vi "Real 64 Converter.vi"(7 "Byte Order (Normal)":T1(ring), 9 "Data In":string) -> (1 "Data Array Out":dbl[](array[numeric]))   [LabVIEW 2017, in "Keithley 2600 Series.lvlib"]
doc: "The KE26XXA_Real64Converter accepts REAL64 double precision IEEE-754 binary formatted data returned by printbuffer() and type casts it to an array of floating point numbers used for data analysis. \n\nEach buffer starts with 2330 and ends with 0A. Everything between is data."
uses:
  Keithley 2600 Series.lvlib
panel:
  out "error out":errorcluster
  in  "error in (no error)":errorcluster
  # "(c) 2008 Keithley Instruments, Inc.  ALL RIGHTS RESERVED."
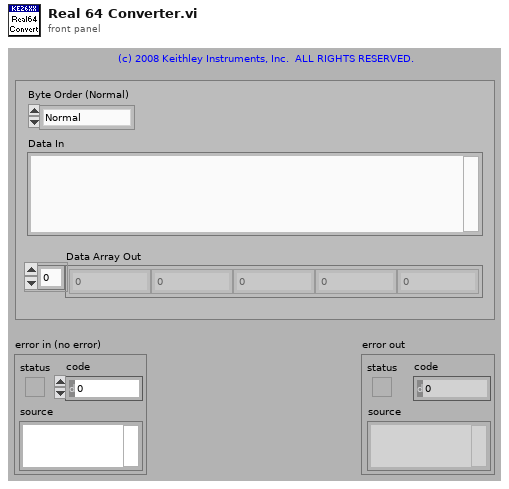
[diagram p1: front panel]
types:
  T1 = enum32{"Normal", "Big Endian", "Little Endian", "Network", "Swapped"}
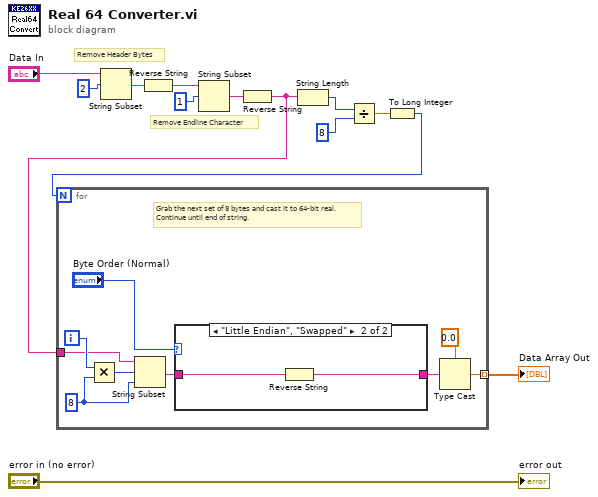
[diagram p0: block diagram]
diagram:
  # "Remove Endline Character"
  # "Remove Header Bytes"
  n1 = String Subset(string="Data In", offset (0)=2) -> (substring=w8:string)  [unwired: 1 out]
  n2 = Reverse String(1:w8) -> (0:w7:string)
  n3 = String Subset(string=w7, offset (0)=1) -> (substring=w5:string)  [unwired: 1 out]
  n4 = Reverse String(1:w5) -> (0:w3:string)
  n5 = String Length(string=w3) -> (length=w12:i32)
  n6 = Divide(x=w12, y=8) -> (x/y=w2:dbl)
  n7 = To Long Integer(number=w2) -> (32bit integer=w1:i32)
  n8 = for {
    N: w1 -> [_]
    tunnel: w3 -> [w16]
    tunnel: [w15] -> w10 mode=indexing
    i -> [w17]
    w18 = 8 ("length (rest)")
    # "Grab the next set of 8 bytes and cast it to 64-bit real.\nContinue until end of string."
    n9 = Multiply(x=w17, y=w18) -> (x*y=w19:i32)
    n10 = String Subset(string=w16, offset (0)=w19, length (rest)=w18) -> (substring=w21:string)
    n11 = case shown="\"Little Endian\", \"Swapped\"" "Byte Order (Normal)" {
      tunnel: w21 -> [w23 w25]
      tunnel: [w23 w24] -> w20
      frame "Normal", "Big Endian", "Network", Default {
      }
      frame "Little Endian", "Swapped" {
        n12 = Reverse String(1:w25) -> (0:w24:string)
      }
    }
    n13 = Type Cast(type=0.0, x=w20) -> (*(type *) &x=w15:dbl)
  }
  "Data Array Out" <- w10
  "error out" <- "error in (no error)"
